vi "Page_Version_Initialize.vi"(6 "output cluster":T1, 8 "error in (no error)":errorcluster, 11 "AB_PackedLibrary in":refnum<class "AB_PackedLibrary.lvclass">) -> (0 "error out":errorcluster, 3 "AB_PackedLibrary out":refnum<class "AB_PackedLibrary.lvclass">)   [LabVIEW 2020, in "AB_PackedLibrary.lvclass"]
uses:
  <vilib>/AppBuilder/AB_Classes/PackedLib/AB_PackedLibrary.lvclass
  <resource>/Framework/Providers/Builds/AppBuilder/AB_UI_Page_Version_References.ctl
  <vilib>/AppBuilder/AB_Classes/TargetFile/AB_Targetfile.lvclass
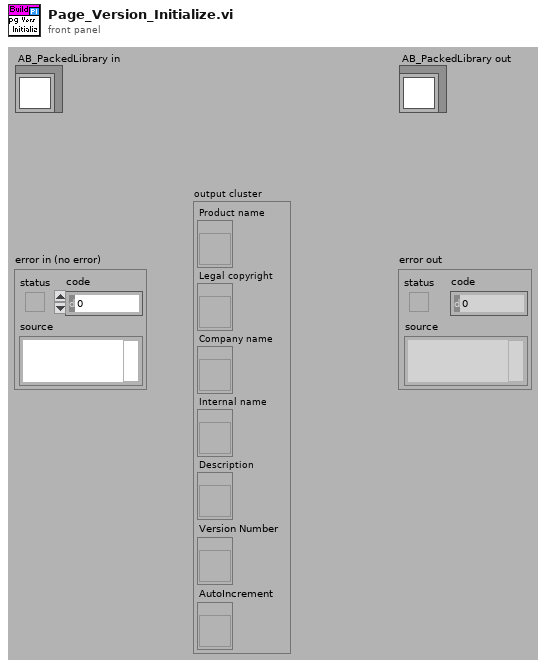
[diagram p1: front panel]
types:
  T1 = typedef "AB_UI_Page_Version_References.ctl" = cluster{"Product name":refnum<vi>, "Legal copyright":refnum<vi>, "Company name":refnum<vi>, "Internal name":refnum<vi>, "Description":refnum<vi>, "Version Number":refnum<vi>, "AutoIncrement":refnum<vi>}
  T2 = enum32{"invalid OS target", "Mac OS", "Windows 3.1", "Windows 95/NT", "Solaris 1", "Solaris 2", "HP-UX", "PowerMAX", "Linux", "Irix", "Rhapsody", "BeOS", "AIX", "OSF1", "VxWorks", "PharLap", "Carbon", "RTX", "Windows x64", "Linux x64", "Mac OS X x64"}
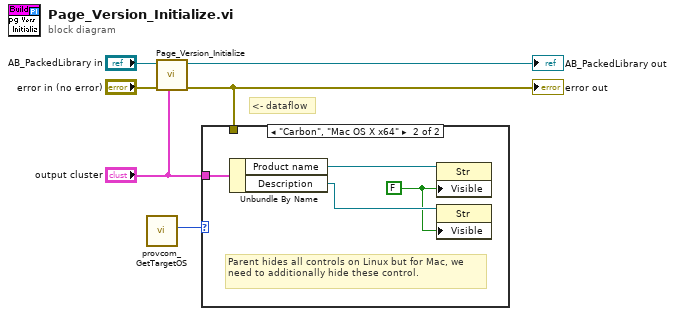
[diagram p0: block diagram]
diagram:
  # "<- dataflow"
  n1 = call <resource>:"provcom_GetTargetOS.vi"() -> ("App.TargetOS"=w3:T2)  [unwired: 11 in]
  n2 = call-parent "Page_Version_Initialize.vi"("output cluster"="output cluster", "error in (no error)"="error in (no error)", "AB_Targetfile in"="AB_PackedLibrary in") -> ("error out"=w1:errorcluster, "AB_Targetfile out"=→"AB_PackedLibrary out":refnum<class "AB_PackedLibrary.lvclass">)  [unwired: 7 in]
  "error out" <- w1
  n3 = case shown="\"Carbon\", \"Mac OS X x64\"" w3 {
    tunnel: "output cluster" -> [_ w10]
    tunnel: w1 -> [_ _]
    frame Default {
    }
    frame "Carbon", "Mac OS X x64" {
      w7 = FALSE ("Visible")
      # "Parent hides all controls on Linux but for Mac, we need to additionally hide these control."
      n4 = Unbundle By Name(w10) -> ("Product name"=w9:refnum<vi>, "Description"=w8:refnum<vi>)
      n5 = property class="Str"(reference=w9, "Visible"=w7) -> ()  [unwired: 1 in, 2 out]
      n6 = property class="Str"(reference=w8, "Visible"=w7) -> ()  [unwired: 1 in, 2 out]
    }
  }
